vi "Make GET Object Request Parameters.vi"(11 "GET Object Request Parameters":T2) -> (3 "HTTP Headers":T1[](array[typedef]))   [LabVIEW 2015, in "NI_AWS_S3.lvlib" / "Object.lvlib"]
uses:
  Object.lvlib
  GET Object Request Parameters.ctl
  Core/Request Range.ctl
  Core/HTTP Request/Name Value Pair.ctl
  Core/HTTP Request/HTTP Request.lvclass
  Core/NI_AWS_Core.lvlib
  NI_AWS_S3.lvlib
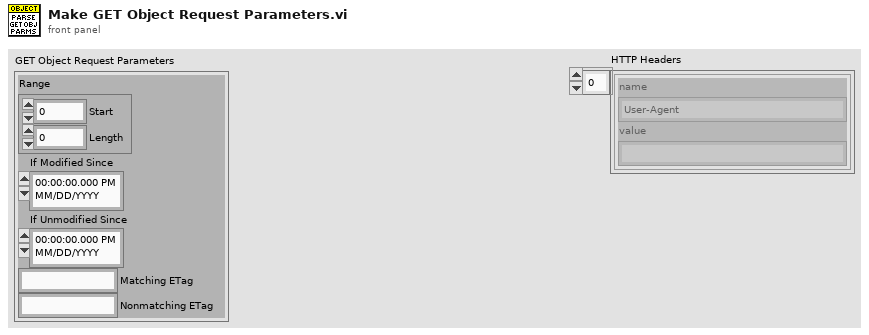
[diagram p1: front panel]
types:
  T1 = typedef "NI_AWS_Core.lvlib/HTTP Request.lvclass/Name Value Pair.ctl" = cluster{"name":string, "value":string}
  T2 = typedef "NI_AWS_S3.lvlib/GET Object Request Parameters.ctl" = cluster{"Range":T3, "If Modified Since":timestamp, "If Unmodified Since":timestamp, "Matching ETag":string, "Nonmatching ETag":string}
  T3 = typedef "NI_AWS_Core.lvlib/Request Range.ctl" = cluster{"Start":i64, "Length":i64}
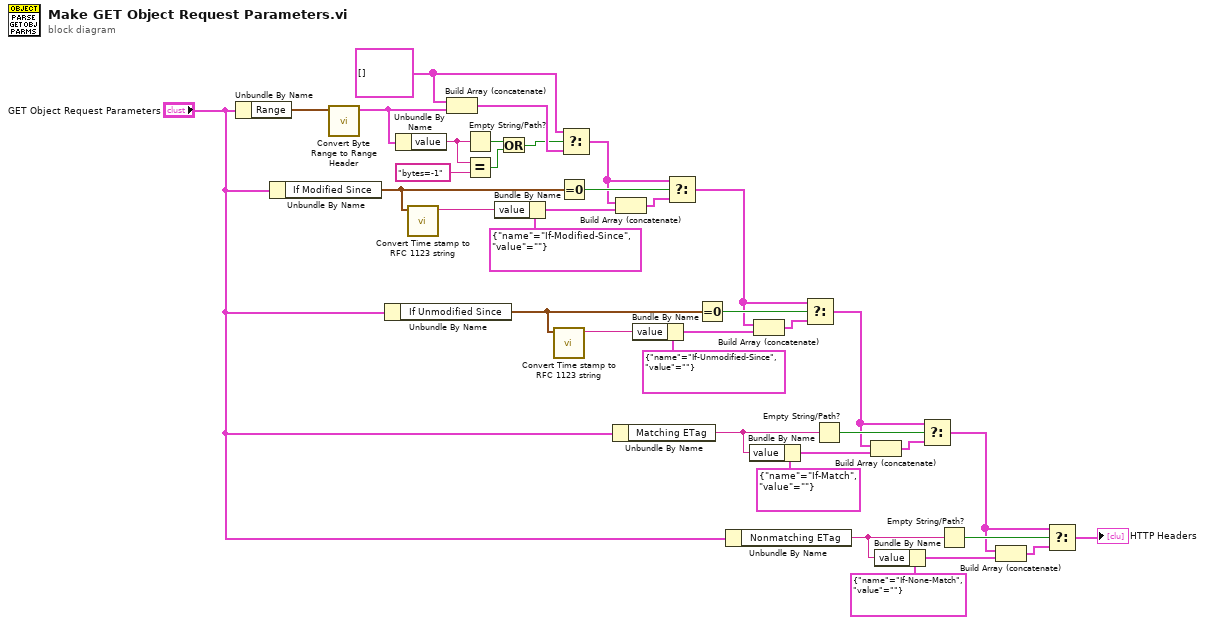
[diagram p0: block diagram]
diagram:
  w1 = T1[] [] ("s? t:f")
  n1 = Unbundle By Name("GET Object Request Parameters") -> ("Range"=w37:T3)
  n2 = Unbundle By Name("GET Object Request Parameters") -> ("If Modified Since"=w28:timestamp)
  n3 = call "Convert Byte Range to Range Header.vi"("Range"=w37) -> ("Range Header"=w36:T1)  [unwired: 10 in]
  n4 = Unbundle By Name("GET Object Request Parameters") -> ("If Unmodified Since"=w27:timestamp)
  n5 = Unbundle By Name(w36) -> ("value"=w6:string)
  n6 = call "Convert Time stamp to RFC 1123 string.vi"("Time Stamp"=w28) -> ("Date Time String (RFC-1123)"=w32:string)  [unwired: 10 in]
  n7 = Build Array (concatenate)(w1, w36) -> (w35:T1[])
  n8 = Empty String/Path?(string/path=w6) -> (empty?=w3:bool)
  n9 = Equal?(x=w6, y="bytes=-1") -> (x = y?=w4:bool)
  n10 = Bundle By Name(cluster=T1 {"name"="If-Modified-Since", "value"=""} ("Name Value Pair"), "value"=w32) -> (w30:T1)
  n11 = Or(x=w3, y=w4) -> (x .or. y?=w2:bool)
  n12 = call "Convert Time stamp to RFC 1123 string.vi"("Time Stamp"=w27) -> ("Date Time String (RFC-1123)"=w24:string)  [unwired: 10 in]
  n13 = Equal To 0?(x=w28) -> (x = 0?=w34:bool)
  n14 = Select(t=w1, s=w2, f=w35) -> (s? t:f=w31:T1[])
  n15 = Unbundle By Name("GET Object Request Parameters") -> ("Matching ETag"=w15:string)
  n16 = Build Array (concatenate)(w31, w30) -> (w29:T1[])
  n17 = Bundle By Name(cluster=T1 {"name"="If-Unmodified-Since", "value"=""} ("Name Value Pair"), "value"=w24) -> (w25:T1)
  n18 = Select(t=w31, s=w34, f=w29) -> (s? t:f=w21:T1[])
  n19 = Equal To 0?(x=w27) -> (x = 0?=w22:bool)
  n20 = Unbundle By Name("GET Object Request Parameters") -> ("Nonmatching ETag"=w14:string)
  n21 = Bundle By Name(cluster=T1 {"name"="If-Match", "value"=""} ("Name Value Pair"), "value"=w15) -> (w18:T1)
  n22 = Build Array (concatenate)(w21, w25) -> (w26:T1[])
  n23 = Select(t=w21, s=w22, f=w26) -> (s? t:f=w16:T1[])
  n24 = Empty String/Path?(string/path=w15) -> (empty?=w20:bool)
  n25 = Build Array (concatenate)(w16, w18) -> (w17:T1[])
  n26 = Bundle By Name(cluster=T1 {"name"="If-None-Match", "value"=""} ("Name Value Pair"), "value"=w14) -> (w12:T1)
  n27 = Select(t=w16, s=w20, f=w17) -> (s? t:f=w9:T1[])
  n28 = Empty String/Path?(string/path=w14) -> (empty?=w10:bool)
  n29 = Build Array (concatenate)(w9, w12) -> (w13:T1[])
  n30 = Select(t=w9, s=w10, f=w13) -> (s? t:f=→"HTTP Headers":T1[])
